vi "main_ctrl.vi"(8 "error in":errorcluster) -> (0 "error out":errorcluster caption="Error")   [LabVIEW 2013]
uses:
  <vilib>/Rock Robotics/WPI/DriverStation/WPI_DriverStationRobotMode2.ctl
  typedefs/Test/test data.ctl
  typedefs/Test/test controls.ctl
  typedefs/fg_typedef.ctl
  typedefs/Vision/vision enable.ctl
  typedefs/Vision/vision data.ctl
  typedefs/State Machine/subStates.ctl
  typedefs/State Machine/singleUseSubstate.ctl
  <vilib>/Rock Robotics/WPI/Solenoid/WPI_SolenoidValue.ctl
  <vilib>/Rock Robotics/WPI/Compressor/WPI_CompressorGetSetRefNum.vi
  <vilib>/Rock Robotics/WPI/RobotDrive/WPI_RobotDriveGetSetRefNum.vi
  <vilib>/Rock Robotics/WPI/RobotDrive/WPI_RobotDriveArcadeDrive_Standard(NoSaturation).vi
  <vilib>/Rock Robotics/WPI/Solenoid/WPI_SolenoidSetEnum.vi
  state machine master/Cancel State Machine - Pickup.vi
  state machine master/Cancel State Machine - Load.vi
panel:
  out "vision errors":errorcluster
  in  "Test\nControls":T1={"Drive Train"=0.0, "Arm"=0.0, "Belts"=0.0, "Drive Train"=FALSE, "Arm"=FALSE, "Belts"=FALSE, "Home Arm Encoder"=FALSE, "Home Right Drive Encoder"=FALSE, "Home Left Drive Encoder"=FALSE, "Extend Shooter"=FALSE, "Retract Shooter"=FALSE, "Latch"=FALSE, "Unlatch"=FALSE, "Shift High"=FALSE, "Shift Low"=FALSE, "Compressor"=TRUE} {"Belts" scale=-1.0..1.0; "Arm" scale=-1.0..1.0; "Drive Train" scale=-1.0..1.0}
  out "Test Data":T2={"Light Sensor"=FALSE, "Shooter Up"=TRUE, "Shooter Down"=FALSE, "Left Rate"=0.0, "Left Distance"=0.0, "Right Rate"=0.0, "Right Distance"=0.0, "Rate"=0.0, "Distance"=0.0, "At Distance Limit"=FALSE, "Encoder Failure"=FALSE, "No Rate Read"=FALSE, "Directional Issue"=FALSE, "Latched"=FALSE, "Unlatched"=TRUE, "Shifted High"=FALSE, "Shifted Low"=TRUE, "Extended"=FALSE, "Retracted"=TRUE, "Left - Encoder Failure"=FALSE, "Left - No Rate Read"=FALSE, "Right - Encoder Failure"=FALSE, "Right - No Rate Read"=FALSE, "Charging"=FALSE, "Full"=FALSE, "On/Off"=FALSE, "DisVision"=FALSE, "2 Ball"=FALSE, "HotGoal"=FALSE, "Shoot"=FALSE}
  out "Robot Mode":T3
  out "Vision mSPI":u32
  out "Vision IPS":dbl
  out "Main IPS":dbl
  out "Main mSPI":u32
  # "Test Input/Output"
  # "MAIN CONTROL"
  # "holds robot control code - dual parallel state machine"
  # "SPI: milliseconds per iteration\nIPS: iterations per second"
  # "Pneumatics"
  # "Home Encoders"
  # "Manual Override"
  # "Joystick Control"
  # "Arm Safeties"
  # "Drive Safeties"
  # "Sensors"
  # "Drive Encoders"
  # "Pneumatics Commands"
  # "Compressor"
  # "Auto Config"
  # "Arm Encoder"
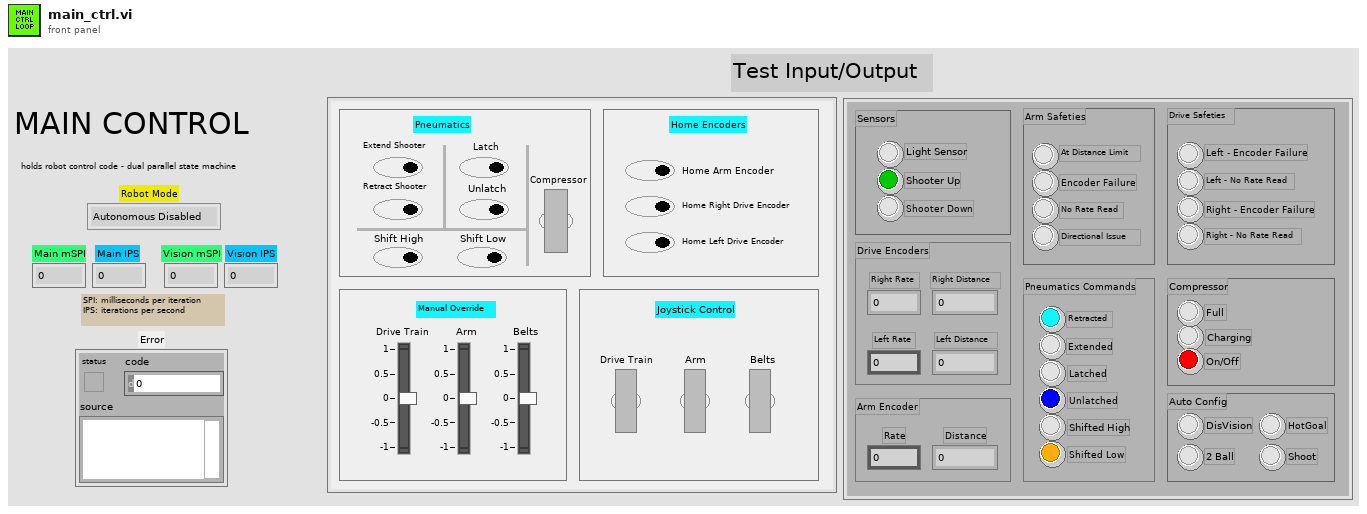
[diagram p1: front panel]
types:
  T1 = typedef "test controls.ctl" = cluster{"Drive Train":dbl, "Arm":dbl, "Belts":dbl, "Drive Train":bool, "Arm":bool, "Belts":bool, "Home Arm Encoder":bool, "Home Right Drive Encoder":bool, "Home Left Drive Encoder":bool, "Extend Shooter":bool, "Retract Shooter":bool, "Latch":bool, "Unlatch":bool, "Shift High":bool, "Shift Low":bool, "Compressor":bool}
  T2 = typedef "test data.ctl" = cluster{"Light Sensor":bool, "Shooter Up":bool, "Shooter Down":bool, "Left Rate":dbl, "Left Distance":dbl, "Right Rate":dbl, "Right Distance":dbl, "Rate":dbl, "Distance":dbl, "At Distance Limit":bool, "Encoder Failure":bool, "No Rate Read":bool, "Directional Issue":bool, "Latched":bool, "Unlatched":bool, "Shifted High":bool, "Shifted Low":bool, "Extended":bool, "Retracted":bool, "Left - Encoder Failure":bool, "Left - No Rate Read":bool, "Right - Encoder Failure":bool, "Right - No Rate Read":bool, "Charging":bool, "Full":bool, "On/Off":bool, "DisVision":bool, "2 Ball":bool, "HotGoal":bool, "Shoot":bool}
  T3 = typedef "WPI_DriverStationRobotMode2.ctl" = enum16{"Autonomous Disabled", "Autonomous Enabled", "Teleop Disabled", "Teleop Enabled", "Timeout", "Finish", "Test Disabled", "Test Enabled"}
  T4 = typedef "fg_typedef.ctl" = enum16{"Get", "Set"}
  T5 = typedef "vision data.ctl" = cluster{"x":dbl, "y":dbl, "area":dbl, "width":dbl, "height":dbl, "Hot Goal Present?":bool, "distance":dbl}
  T6 = typedef "vision enable.ctl" = enum16{"Enable", "Disable", "Stop"}
  T7 = typedef "WPI_CameraDevRef.ctl" = cluster{"Camera Address":string, "CameraStatus":errorcluster, "Acquire Image Notifier":refnum<notifier>}
  T8 = typedef "IMAQ Image.ctl" = refnum<image>
  T9 = cluster{"Vision mSPI":u32, "Main mSPI":u32, "Dash mSPI":u32}
  T10 = typedef "WPI_RobotDriveDevRef.ctl" = cluster{"DevStatus":errorcluster, "Motors[]":T11[], "Square Inputs":bool, "Max Output":dbl, "Isochronous":bool}
  T11 = typedef "WPI_MotorControlDeviceRef.ctl" = cluster{"DeviceStatus":errorcluster, "Type":enum16{"PWM", "CAN"}, "PWM":cluster{"Digital Module":T12, "PWM Channel":T13, "DeadBand":T14}, "CAN":cluster{"Device Number":u8, "Control Mode":T15, "Semaphore":T16, "Max Vout":dbl}, "Invert":bool, "TransformRef":T17, "InvTransformRef":T17}
  T12 = typedef "FPGA_TypedefDigitalModule.ctl" = enum16{"Digital Module 1", "Digital Module 2"}
  T13 = typedef "FPGA_DIOPWMChannel.ctl" = enum8{"PWM 1", "PWM 2", "PWM 3", "PWM 4", "PWM 5", "PWM 6", "PWM 7", "PWM 8", "PWM 9", "PWM 10", "Invalid"}
  T14 = typedef "WPI_PWMDeadband.ctl" = cluster{"Name":string, "maxPositivePwm":i32, "minPositivePwm":i32, "centerPwm":i32, "maxNegativePwm":i32, "minNegativePwm":i32, "angularRange":u16}
  T15 = typedef "WPI_CANJaguar_ControlMode.ctl" = enum8{"Percent VBus", "Current", "Speed", "Position", "Voltage"}
  T16 = typedef "Semaphore RefNum" = refnum<k1>
  T17 = typedef "WPI_PWMTransform_ConPane.ctl" = refnum<vi>
  T18 = typedef "WPI_SolenoidDevRef.ctl" = cluster{"DevStatus":errorcluster, "Solenoid Module":T19, "Forward Solenoid Channel":T20, "Reverse Solenoid Channel":T20}
  T19 = typedef "FPGA_TypedefSolenoidModule.ctl" = enum16{"Solenoid Module 1", "Solenoid Module 2"}
  T20 = typedef "WPI_SolenoidChannel.ctl" = enum8{"Solenoid 1", "Solenoid 2", "Solenoid 3", "Solenoid 4", "Solenoid 5", "Solenoid 6", "Solenoid 7", "Solenoid 8", "Invalid"}
  T21 = typedef "WPI_CompressorDevRef.ctl" = cluster{"DevStatus":errorcluster, "DigitalInputDevRef":T22, "RelayDevRef":T24}
  T22 = typedef "WPI_DigitalInputDevRef.ctl" = cluster{"DevStatus":errorcluster, "DIO Channel":T23, "Digital Module":T12}
  T23 = typedef "FPGA_DIOChannel.ctl" = enum8{"DIO 1", "DIO 2", "DIO 3", "DIO 4", "DIO 5", "DIO 6", "DIO 7", "DIO 8", "DIO 9", "DIO 10", "DIO 11", "DIO 12", "DIO 13", "DIO 14", "Invalid"}
  T24 = typedef "WPI_RelayDevRef.ctl" = cluster{"DevStatus":errorcluster, "Relay Channel":T25, "Digital Module":T12, "Relay Direction":T26}
  T25 = typedef "FPGA_DIORelayChannel.ctl" = enum8{"Relay 1", "Relay 2", "Relay 3", "Relay 4", "Relay 5", "Relay 6", "Relay 7", "Relay 8", "Invalid"}
  T26 = typedef "WPI_RelayDirection.ctl" = enum16{"Both directions", "Forward only", "Reverse only"}
  T27 = typedef "WPI_SolenoidValue.ctl" = enum16{"Off", "On", "Forward", "Reverse"}
  T28 = typedef "subStates.ctl" = enum16{"null", "wait", "driver control", "auto", "manual override", "hold position", "rotate", "pickup", "pass", "recover pass", "load", "goto shoot", "shoot high goal", "shoot low goal", "cancel arm", "cancel shooter", "end", "test"}
  T29 = typedef "singleUseSubstate.ctl" = enum16{"null", "wait", "shift high", "shift low", "extend shooter", "retract shooter", "latch", "unlatch", "end"}
  T30 = typedef "WPI_DriverStationMatch Info.ctl" = cluster{"Autonomous Elapsed Seconds":dbl, "TeleOp Elapsed Seconds":dbl, "Disabled Elapsed Seconds":dbl, "Visited Autonomous":bool, "Visited TeleOp":bool, "Visited Disabled":bool, "Autonomous Settings":cluster{"Autonomous Style":enum16{"Iterative", "Independent"}, "VI Refnum":refnum<vi>}}
  T31 = typedef "WPI_DriverStationDerivedRobotMode.ctl" = enum16{"Init", "Execute", "Stop"}
  T32 = typedef "Loop 2 Datatype.ctl" = cluster{"State":T28, "Waiting Loop":i32, "State to Wait For":i32, "Loop ID":i32, "Exit Value":i32, "Joystick Y":dbl, "Joystick Z":dbl}
  T33 = typedef "Loop 1 Datatype.ctl" = cluster{"State":T28, "Waiting Loop":i32, "State to Wait For":i32, "Loop ID":i32, "Exit Value":i32}
  T34 = typedef "Loop 3 Datatype.ctl" = cluster{"State":T28, "Waiting Loop":i32, "State to Wait For":i32, "Loop ID":i32, "Exit Value":i32, "Joystick Y":dbl, "Tune Setpoint":cluster{"Increment":bool, "Decrement":bool}}
  T35 = typedef "Loop 0 Datatype.ctl" = cluster{"State":T28, "Waiting Loop":i32, "State to Wait For":i32, "Loop ID":i32, "Exit Value":i32, "X Axis":dbl, "Y Axis":dbl, "Z Axis":dbl}
  T36 = typedef "dashboard safety status data.ctl" = cluster{"At Distance Limit":bool, "No Rate Read":bool, "Encoder Failure":bool, "Encoder Directional Issue":bool}
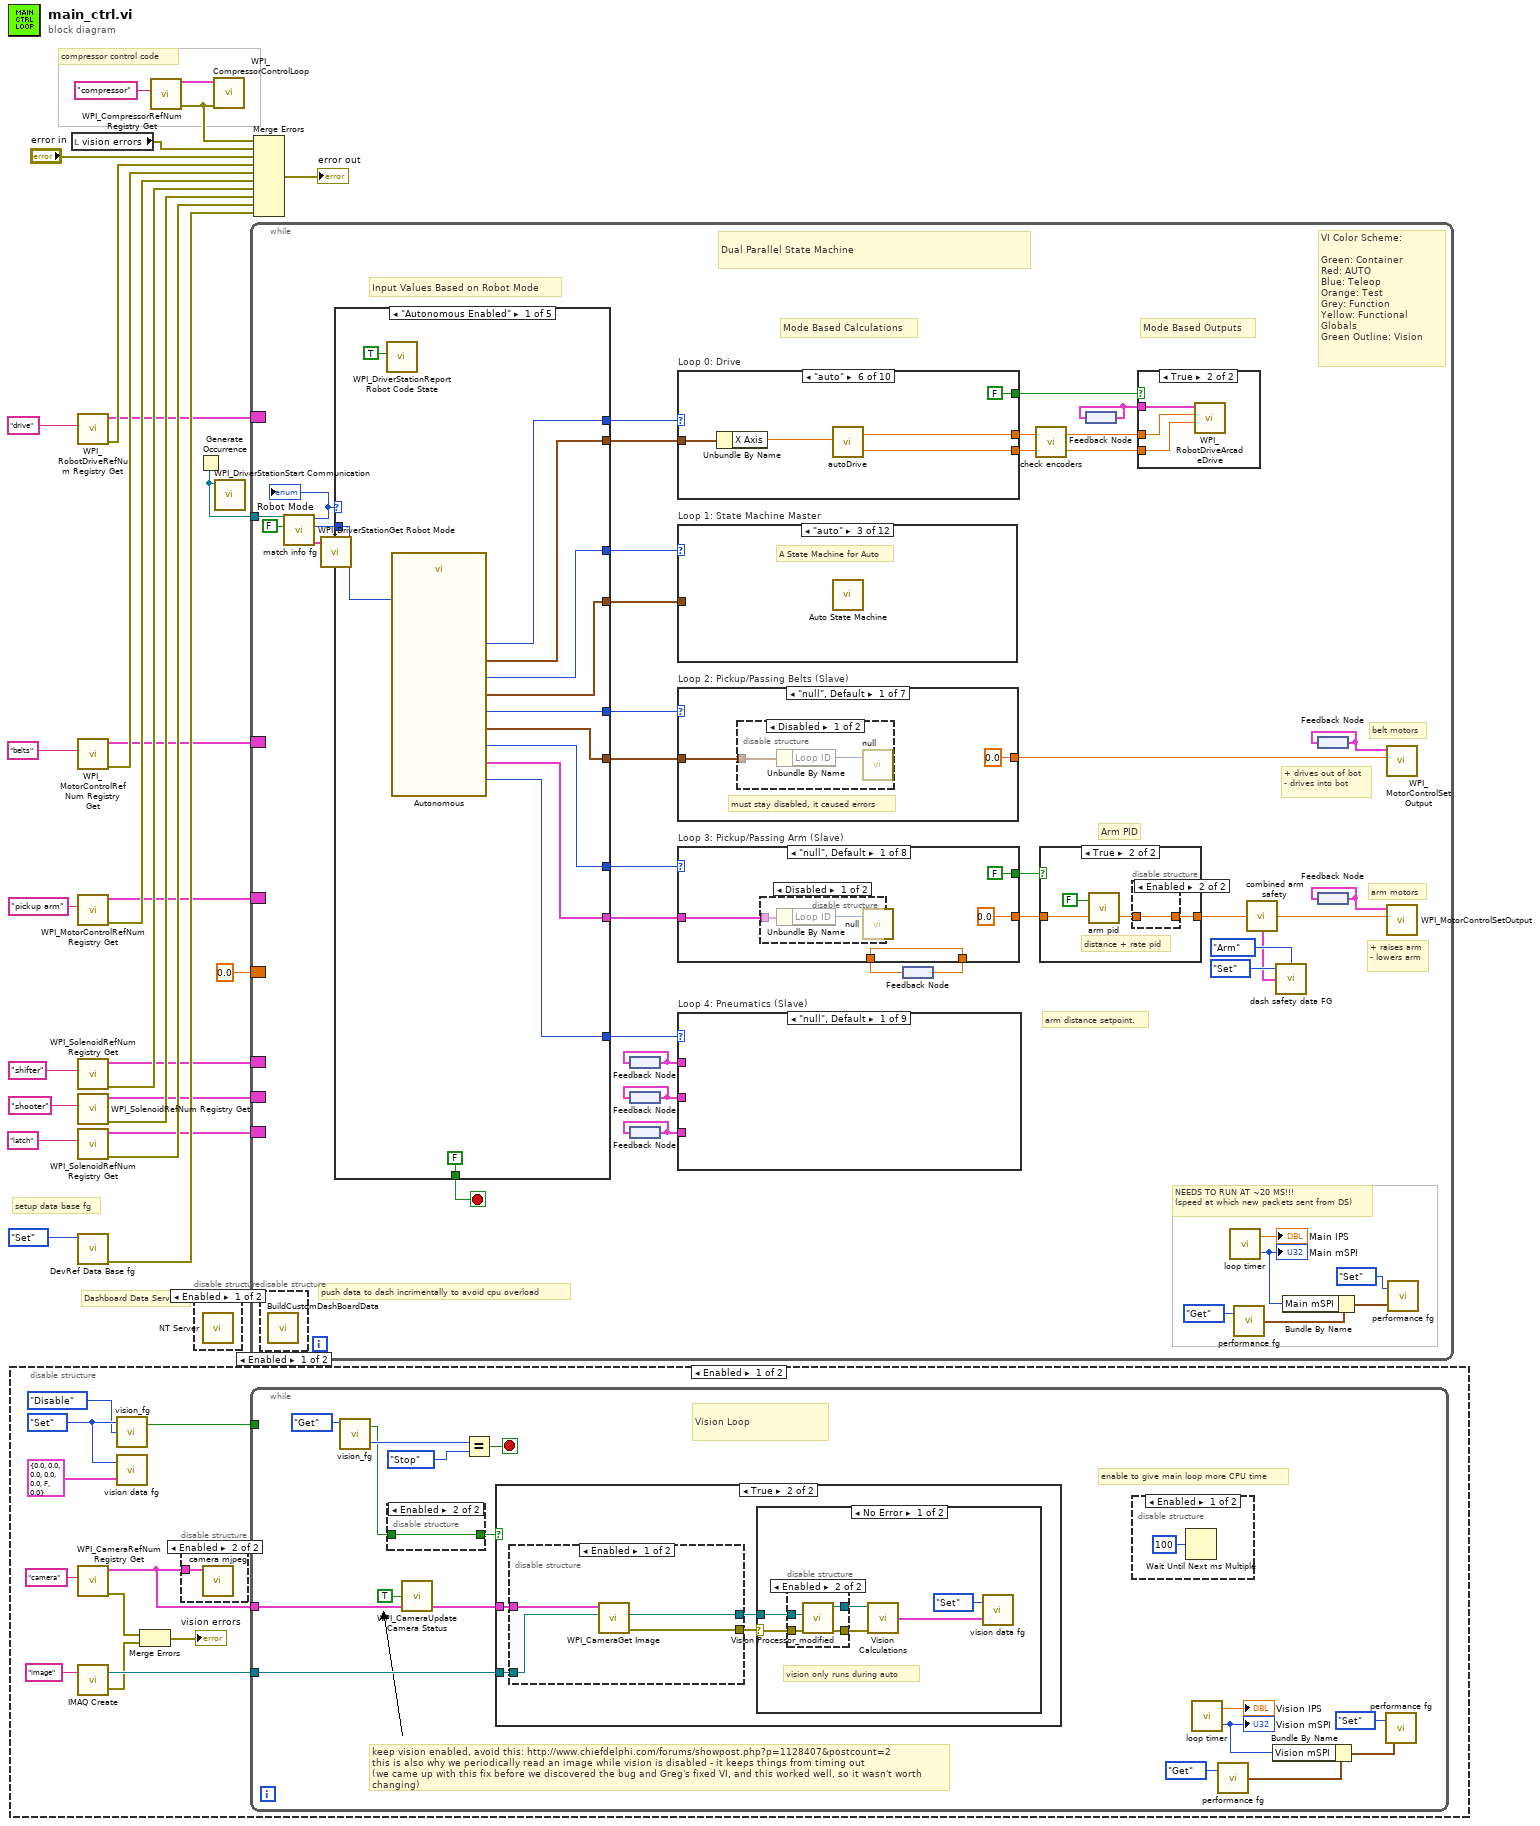
[diagram p0: block diagram]
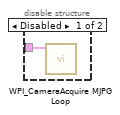
[diagram p3: hidden frame]
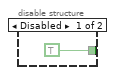
[diagram p4: hidden frame]
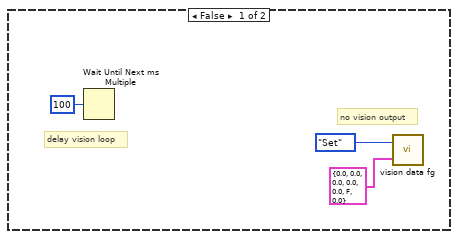
[diagram p6: hidden frame]
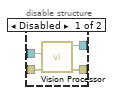
[diagram p7: hidden frame]
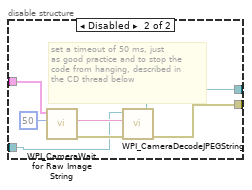
[diagram p9: hidden frame]
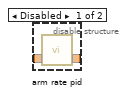
[diagram p12: hidden frame]
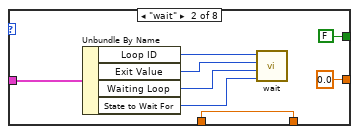
[diagram p14: hidden frame]
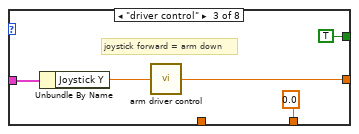
[diagram p15: hidden frame]
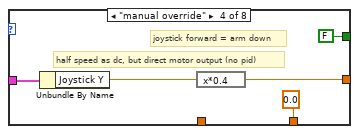
[diagram p16: hidden frame]
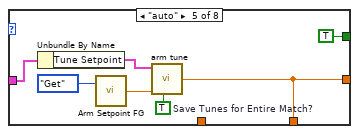
[diagram p17: hidden frame]
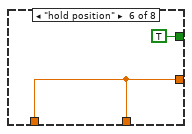
[diagram p18: hidden frame]
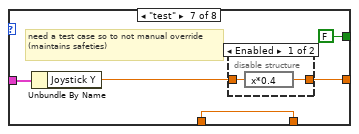
[diagram p19: hidden frame]
diagram:
  # "compressor control code"
  # "Dashboard Data Server"
  # "setup data base fg"
  n1 = disable-structure shown="Enabled" {
    frame Enabled {
      w37 = fg_typedef."Set" ("Enum")
      n2 = call <vilib>:"WPI_CameraRefNum Registry Get.vi"("refnum name"="camera") -> ("error out"=w30:errorcluster, "CameraDevRef"=w34:T7)  [unwired: 9 in]
      n3 = call "IMAQ Create"("Image Name"="image") -> ("New Image"=w39:T8, "error out"=w31:errorcluster)  [unwired: 4 in]
      n4 = call "vision_fg.vi"("Action"=vision_enable."Disable", "Menu"=w37) -> ("Enabled?"=w38:bool)  [unwired: 1 in, 1 out]
      n5 = call "vision data fg.vi"("Input"=T5 {"x"=0.0, "y"=0.0, "area"=0.0, "width"=0.0, "height"=0.0, "Hot Goal Present?"=FALSE, "distance"=0.0} ("Cluster"), "Menu"=w37) -> ()  [unwired: 1 out]
      n6 = Merge Errors(w30, w31) -> (→"vision errors":errorcluster)
      n7 = disable-structure shown="Enabled" {
        disable-tunnel: w34 -> [w40 w41]
        frame Disabled {
          n8 = call <vilib>:"WPI_CameraAcquire MJPG Loop.vi"("CameraDevRef"=w40) -> ()  [unwired: 11 in]
        }
        frame Enabled {
          n9 = call "camera mjpeg.vi"("CameraDevRef"=w41) -> ()  [unwired: 11 in]
        }
      }
      n10 = while {
        tunnel: w39 -> [w56]
        tunnel: w34 -> [w55]
        tunnel: w38 -> [_]
        stop <- w57 stop-if-true
        # "keep vision enabled, avoid this: http://www.chiefdelphi.com/forums/showpost.php?p=1128407&postcount=2\nthis is also why we periodically read an image while vision is disabled - it keeps things from timing out\n(we came up with this fix before we discovered the bug and Greg's fixed VI, and this worked well, so it wasn't worth changing)"
        # "enable to give main loop more CPU time"
        # "Vision Loop"
        n11 = call "vision_fg.vi"("Menu"=fg_typedef."Get" ("Enum")) -> ("State Out"=w51:T6, "Enabled?"=w42:bool)  [unwired: 2 in]
        n12 = disable-structure shown="Enabled" {
          disable-tunnel: [TRUE w59] -> w43
          disable-tunnel: w42 -> [_ w59]
          frame Disabled {
          }
          frame Enabled {
          }
        }
        n13 = call <vilib>:"WPI_CameraUpdate Camera Status.vi"("CameraDevRef In"=w55, "Enable Vision"=TRUE) -> ("CameraDevRef Out"=w54:T7)  [unwired: 3 in]
        n14 = Equal?(x=w51, y=vision_enable."Stop") -> (x = y?=w57:bool)
        n15 = case shown="True" w43 {
          tunnel: w56 -> [_ w67]
          tunnel: w54 -> [_ w66]
          frame False {
            # "no vision output"
            # "delay vision loop"
            n16 = Wait Until Next ms Multiple(millisecond multiple=u32 100) -> ()  [unwired: 1 out]
            n17 = call "vision data fg.vi"("Input"=T5 {"x"=0.0, "y"=0.0, "area"=0.0, "width"=0.0, "height"=0.0, "Hot Goal Present?"=FALSE, "distance"=0.0} ("Cluster"), "Menu"=fg_typedef."Set" ("Enum")) -> ()  [unwired: 1 out]
          }
          frame True {
            n18 = disable-structure shown="Enabled" {
              disable-tunnel: w67 -> [w84 w88]
              disable-tunnel: w66 -> [w85 w90]
              disable-tunnel: [w83 w87] -> w65
              disable-tunnel: [w82 w86] -> w64
              frame Enabled {
                n19 = call <vilib>:"WPI_CameraGet Image.vi"("Image"=w84, "CameraDevRef"=w85) -> ("error out"=w82:errorcluster, "Image Out"=w83:T8)  [unwired: 7 in, 1 out]
              }
              frame Disabled {
                # "set a timeout of 50 ms, just\nas good practice and to stop the \ncode from hanging, described in \nthe CD thread below"
                n20 = call <vilib>:"WPI_CameraWait for Raw Image String.vi"("Timeout in ms (-1)"=50, "CameraDevRef"=w90) -> ("error out"=w92:errorcluster, "String"=w91:string)  [unwired: 3 in, 5 out]
                n21 = call <vilib>:"WPI_CameraDecodeJPEGString.vi"("error in"=w92, "Compressed Image"=w91, "Image In"=w88) -> ("error out"=w86:errorcluster, "Image Out"=w87:T8)  [unwired: 3 out]
              }
            }
            n22 = case shown="No Error" w64 {
              selector: w64 -> [w72 _]
              tunnel: w65 -> [w71 _]
              frame No Error {
                # "vision only runs during auto"
                n23 = disable-structure shown="Enabled" {
                  disable-tunnel: w72 -> [w77 w80]
                  disable-tunnel: w71 -> [w76 w81]
                  disable-tunnel: [w75 w78] -> w70
                  disable-tunnel: [w74 w79] -> w69
                  frame Disabled {
                    n24 = call "Vision Processor.vi"("error in"=w77, "Image In"=w76) -> ("error out"=w74:errorcluster, "Image Out"=w75:T8)  [unwired: 5 in]
                  }
                  frame Enabled {
                    n25 = call "Vision Processor_modified.vi"("error in"=w80, "Image In"=w81) -> ("error out"=w79:errorcluster, "Image Out"=w78:T8)  [unwired: 5 in]
                  }
                }
                n26 = call "Vision Calculations.vi"("Image In"=w70, "error in"=w69) -> ("Vision Data"=w68:T5)  [unwired: 3 in]
                n27 = call "vision data fg.vi"("Input"=w68, "Menu"=fg_typedef."Set" ("Enum")) -> ()  [unwired: 1 out]
              }
              frame Error {
              }
            }
          }
        }
        n28 = disable-structure shown="Enabled" {
          frame Enabled {
            n29 = Wait Until Next ms Multiple(millisecond multiple=u32 100) -> ()  [unwired: 1 out]
          }
          frame Disabled {
          }
        }
        n30 = call "loop timer.vi"() -> ("IPS"=→"Vision IPS":dbl, "SPI"=w49:u32)  [unwired: 1 in]
        "Vision mSPI" <- w49
        n31 = call "performance fg.vi"("Menu"=fg_typedef."Get") -> ("Output"=w47:T9)  [unwired: 1 in]
        n32 = Bundle By Name(cluster=w47, "Vision mSPI"=w49) -> (w46:T9)
        n33 = call "performance fg.vi"("Input"=w46, "Menu"=fg_typedef."Set") -> ()  [unwired: 1 out]
      }
    }
    frame Disabled {
      # "vision disabled"
    }
  }
  n34 = local read "vision errors"() -> (w1:errorcluster)
  n35 = call <vilib>:"WPI_RobotDriveRefNum Registry Get.vi"("refnum name"="drive") -> ("error out"=w27:errorcluster, "RobotDriveDevRef"=w3:T10)  [unwired: 9 in]
  n36 = call <vilib>:"WPI_MotorControlRefNum Registry Get.vi"("refnum name"="belts") -> ("error out"=w26:errorcluster, "MotorControlDevRef"=w7:T11)  [unwired: 9 in]
  n37 = call <vilib>:"WPI_MotorControlRefNum Registry Get.vi"("refnum name"="pickup arm") -> ("error out"=w25:errorcluster, "MotorControlDevRef"=w10:T11)  [unwired: 9 in]
  n38 = call <vilib>:"WPI_SolenoidRefNum Registry Get.vi"("refnum name"="shifter") -> ("error out"=w24:errorcluster, "SolenoidDevRef"=w17:T18)  [unwired: 9 in]
  n39 = call <vilib>:"WPI_SolenoidRefNum Registry Get.vi"("refnum name"="shooter") -> ("error out"=w23:errorcluster, "SolenoidDevRef"=w5:T18)  [unwired: 9 in]
  n40 = call <vilib>:"WPI_SolenoidRefNum Registry Get.vi"("refnum name"="latch") -> ("error out"=w22:errorcluster, "SolenoidDevRef"=w6:T18)  [unwired: 9 in]
  n41 = call "DevRef Data Base fg.vi"("Menu"=fg_typedef."Set") -> ("error out"=w28:errorcluster)  [unwired: 2 in, 8 out]
  n42 = call <vilib>:"WPI_CompressorRefNum Registry Get.vi"("refnum name"="compressor") -> ("error out"=w2:errorcluster, "CompressorDevRef"=w18:T21)  [unwired: 9 in]
  n43 = disable-structure shown="Enabled" {
    frame Enabled {
      n44 = call <vilib>:"NT Server.vi"() -> ()  [unwired: 12 in]
    }
    frame Disabled {
    }
  }
  n45 = Generate Occurrence() -> (w15:refnum<k4>)
  n46 = call <vilib>:"WPI_CompressorControlLoop.vi"("error in (no error)"=w2, "CompressorDevRef"=w18) -> ()  [unwired: 10 in]
  n47 = call <vilib>:"WPI_DriverStationStart Communication.vi"("occurrence"=w15) -> ()  [unwired: 11 in]
  n48 = while {
    tunnel: w15 -> [w116]
    border: w3 -> [_]
    border: w17 -> [_]
    border: w6 -> [_]
    border: w5 -> [_]
    border: w7 -> [_]
    border: w10 -> [_]
    border: 0.0 ("setpoint") -> [_]
    stop <- w131 stop-if-true
    # "Arm PID"
    # "Mode Based Outputs"
    # "arm motors"
    # "arm distance setpoint."
    # "push data to dash incrimentally to avoid cpu overload"
    # "+ raises arm\n- lowers arm"
    # "+ drives out of bot\n- drives into bot"
    # "belt motors"
    # "VI Color Scheme:\n\nGreen: Container\nRed: AUTO\nBlue: Teleop\nOrange: Test \nGrey: Function\nYellow: Functional Globals\nGreen Outline: Vision"
    # "Input Values Based on Robot Mode"
    # "Mode Based Calculations"
    # "NEEDS TO RUN AT ~20 MS!!!\n(speed at which new packets sent from DS)"
    # "Dual Parallel State Machine"
    n49 = disable-structure shown="Enabled" {
      frame Enabled {
        n50 = call "BuildCustomDashBoardData.vi"() -> ()  [unwired: 12 in]
      }
      frame Disabled {
      }
    }
    n51 = call <vilib>:"WPI_DriverStationGet Robot Mode.vi"("Finish"=FALSE, "DS Occurrence"=w116) -> ("Match Info out"=w99:T30, "Call Context"=w115:T31, "Robot Mode"=w114:T3)  [unwired: 7 out]
    "Robot Mode" <- w114
    n52 = call "match info fg.vi"("Match Info"=w99) -> ()  [unwired: 26 in, 1 out]
    n53 = case shown="\"Autonomous Enabled\"" w114 {
      tunnel: [w321 w336 w345 w353 w359] -> w118
      tunnel: w115 -> [w314 w332 w348 _ _]
      tunnel: [w319 w335 w347 w353 w359] -> w133
      tunnel: [w315 w333 w339 singleUseSubstate."null" ("SubState 5") singleUseSubstate."end" ("SubState 5")] -> w132
      tunnel: [FALSE FALSE FALSE FALSE TRUE] -> w131
      tunnel: [w323 w331 w343 w353 w359] -> w108
      tunnel: [w322 w330 w344 _ _] -> w125
      tunnel: [w320 w329 w346 _ _] -> w124
      tunnel: [w318 w328 w342 _ _] -> w123
      tunnel: [w316 w327 w340 _ _] -> w121
      tunnel: [w317 w326 w341 w353 w359] -> w107
      frame "Autonomous Enabled" {
        n54 = call <vilib>:"WPI_DriverStationReport Robot Code State.vi"("Autonomous"=TRUE) -> ()  [unwired: 10 in, 1 out]
        n55 = call "Autonomous.vi"("Call Context"=w314) -> ("SubState 2"=w319:T28, "Loop 2 Data"=w318:T32, "SubState 1"=w321:T28, "Loop 1 Data"=w320:T33, "Loop 3 Data"=w316:T34, "SubState 0"=w323:T28, "SubState 3"=w317:T28, "Loop 0 Data"=w322:T35, "SubState 4"=w315:T29)  [unwired: 2 in]
      }
      frame "Teleop Enabled" {
        n56 = call <vilib>:"WPI_DriverStationReport Robot Code State.vi"("TeleOp"=TRUE) -> ()  [unwired: 10 in, 1 out]
        n57 = call "Teleop.vi"("Call Context"=w332) -> ("SubState 3"=w326:T28, "SubState 4"=w333:T29, "Loop 3 Data"=w327:T34, "SubState 0"=w331:T28, "Loop 1 Data"=w329:T33, "Loop 0 Data"=w330:T35, "SubState 1"=w336:T28, "Loop 2 Data"=w328:T32, "SubState 2"=w335:T28)  [unwired: 10 in]
      }
      frame "Test Enabled" {
        n58 = call <vilib>:"WPI_DriverStationReport Robot Code State.vi"("Test"=TRUE) -> ()  [unwired: 10 in, 1 out]
        n59 = call "Test.vi"("Test Controls"="Test\nControls", "Call Context"=w348) -> ("Loop 2 Data"=w342:T32, "SubState 2"=w347:T28, "Loop 1 Data"=w346:T33, "SubState 1"=w345:T28, "SubState 3"=w341:T28, "Loop 0 Data"=w344:T35, "Loop 3 Data"=w340:T34, "SubState 0"=w343:T28, "SubState 4"=w339:T29, "Test Data"=→"Test Data":T2)
      }
      frame "Autonomous Disabled", "Teleop Disabled", "Timeout", "Test Disabled" {
        w353 = subStates."null" ("SubState 0")
        # "set all loops to null"
        # "make sure to disable vision\nwe don't need it here"
        # "robot disabled, timeout"
        n60 = call <vilib>:"WPI_DriverStationReport Robot Code State.vi"("Disabled"=TRUE) -> ()  [unwired: 10 in, 1 out]
        n61 = call "vision_fg.vi"("Action"=vision_enable."Disable", "Menu"=fg_typedef."Set") -> ()  [unwired: 1 in, 2 out]
      }
      frame "Finish" {
        w359 = subStates."end" ("Loop State")
        # "Stop All Loops"
        # "stop the while loop"
        # "stop DS comms"
        # "stop vision loop"
        n62 = call <vilib>:"WPI_DriverStationStop Communication.vi"("StopCommunication"=TRUE) -> ()  [unwired: 10 in, 1 out]
        n63 = call "vision_fg.vi"("Action"=vision_enable."Stop", "Menu"=fg_typedef."Set") -> ()  [unwired: 1 in, 2 out]
      }
    }
    n64 = feedback #1() -> (w122:T18)
    n65 = feedback-in #1(w122) -> ()
    n66 = feedback #2() -> (w110:T18)
    n67 = feedback-in #2(w110) -> ()
    n68 = feedback #3() -> (w109:T18)
    n69 = feedback-in #3(w109) -> ()
    n70 = case "Loop 0: Drive" shown="\"auto\"" w108 {
      tunnel: w125 -> [w221 w226 w236 w248 w256 w259 w265 _ w278 _]
      tunnel: [w220 w225 w235 w245 w253 w261 w267 w269 0.0 ("X Axis") w280] -> w96
      tunnel: [w220 w225 w234 w244 w252 w260 w266 w268 w277 w280] -> w95
      tunnel: [FALSE FALSE TRUE FALSE FALSE FALSE FALSE FALSE TRUE FALSE] -> w120
      frame "null", Default {
        w220 = 0.0 ("X Axis")
        n71 = disable-structure shown="Disabled" {
          disable-tunnel: w221 -> [w223 _]
          frame Disabled {
            n72 = Unbundle By Name(w223) -> ("Loop ID"=w222:i32)
            n73 = call "null.vi"("This Loop ID"=w222) -> ()  [unwired: 2 in]
          }
          frame Enabled {
          }
        }
      }
      frame "wait" {
        w225 = 0.0 ("X Axis")
        n74 = Unbundle By Name(w226) -> ("Loop ID"=w230:i32, "Exit Value"=w229:i32, "Waiting Loop"=w228:i32, "State to Wait For"=w227:i32)
        n75 = call "wait.vi"("State to wait for"=w227, "Waiting Loop ID"=w228, "time (ms)"=w229, "Current Loop ID"=w230) -> ()  [unwired: 1 out]
      }
      frame "driver control" {
        n76 = Unbundle By Name(w236) -> ("X Axis"=w232:dbl, "Y Axis"=w233:dbl)
        n77 = disable-structure shown="Enabled" {
          disable-tunnel: w232 -> [w240 w242]
          disable-tunnel: w233 -> [w239 w241]
          disable-tunnel: [w238 w242] -> w235
          disable-tunnel: [w237 w241] -> w234
          frame Disabled {
            n78 = call "calc arcade drive pwm.vi"("Y axis value"=w239, "X axis value"=w240) -> ("Right Speed"=w237:dbl, "Left Speed"=w238:dbl)  [unwired: 1 in, 1 out]
          }
          frame Enabled {
          }
        }
      }
      frame "manual override" {
        n79 = Unbundle By Name(w248) -> ("X Axis"=w247:dbl, "Y Axis"=w246:dbl)
        n80 = expression code="x/2"(w247) -> (w245:dbl)
        n81 = expression code="x/2"(w246) -> (w244:dbl)
      }
      frame "hold position" {
        n82 = Unbundle By Name(w256) -> ("X Axis"=w255:dbl, "Y Axis"=w254:dbl)
        n83 = call "closed drive.vi"("Acrade Drive?"=TRUE, "Y axis value (Left)"=w254, "X axis value (Right)"=w255, "Threshold (.4)"=0.4) -> ("right"=w252:dbl, "left"=w253:dbl)
      }
      frame "auto" {
        n84 = Unbundle By Name(w259) -> ("X Axis"=w257:dbl)
        n85 = call "autoDrive.vi"("Distance"=w257) -> ("right speed"=w260:dbl, "left speed"=w261:dbl)  [unwired: 2 in, 1 out]
      }
      frame "rotate" {
        n86 = Unbundle By Name(w265) -> ("X Axis"=w264:dbl, "Y Axis"=w263:dbl)
        n87 = call "rotate.vi"("Rate"=w263, "Angle"=w264) -> ("right speed"=w266:dbl, "left speed"=w267:dbl)  [unwired: 1 in, 1 out]
      }
      frame "goto shoot" {
        n88 = disable-structure shown="Enabled" {
          disable-tunnel: [w272 _] -> w269
          disable-tunnel: [w271 _] -> w268
          frame Disabled {
            # "consider implimenting closed hold with drive"
            n89 = call "vision data fg.vi"("Menu"=fg_typedef."Get") -> ("Output"=w273:T5)  [unwired: 1 in]
            n90 = call "goto location.vi"("Image Data"=w273) -> ("left speed"=w272:dbl, "right speed"=w271:dbl)
          }
          frame Enabled {
            # "not going to do this"
          }
        }
      }
      frame "test" {
        n91 = Unbundle By Name(w278) -> ("Y Axis"=w277:dbl)
      }
      frame "end" {
        w280 = 0.0 ("X Axis")
      }
    }
    n92 = case "Loop 1: State Machine Master" shown="\"auto\"" w118 {
      tunnel: w124 -> [w298 w299 _ _ _ _ _ _ _ _ _ _]
      frame "null", Default {
        n93 = Unbundle By Name(w298) -> ("Loop ID"=w297:i32)
        n94 = call "null.vi"("This Loop ID"=w297) -> ()  [unwired: 2 in]
      }
      frame "wait" {
        n95 = Unbundle By Name(w299) -> ("Loop ID"=w303:i32, "Exit Value"=w302:i32, "Waiting Loop"=w301:i32, "State to Wait For"=w300:i32)
        n96 = call "wait.vi"("State to wait for"=w300, "Waiting Loop ID"=w301, "time (ms)"=w302, "Current Loop ID"=w303) -> ()  [unwired: 1 out]
      }
      frame "auto" {
        # "A State Machine for Auto"
        n97 = call "Auto State Machine.vi"() -> ()  [unwired: 12 in]
      }
      frame "manual override" {
        w309 = FALSE ("Can Shoot Safely?")
        w304 = TRUE ("exit in")
        # "Manual Shoot"
        n98 = call "single use states FG.vi"("exit in"=w304, "substate"=singleUseSubstate."unlatch", "menu (get)"=enum16{"set", "get"}."set") -> ()  [unwired: 5 in, 4 out]
        n99 = call "states FG.vi"("exit in"=w304, "subState in"=subStates."null", "menu (get)"=enum16{"set", "get"}."set", "Loop ID"=1) -> ()  [unwired: 4 in, 4 out]
        n100 = call "safe shoot error.vi"("Can Shoot Safely?"=w309, "Menu"=fg_typedef."Set") -> ()  [unwired: 1 out]
        n101 = call "arm during load cancel.vi"("Arm Canceled During Load?"=w309, "Mode"=enum16{"Get", "Set", "Teleop Set"}."Set") -> ()  [unwired: 1 out]
      }
      frame "pickup" {
        # "A State Machine for Pickup"
        n102 = call "Pickup State Machine.vi"() -> ()  [unwired: 12 in]
      }
      frame "pass" {
        # "A State Machine for Passing"
        n103 = call "Pass State Machine.vi"() -> ()  [unwired: 12 in]
      }
      frame "recover pass" {
        # "If a pass fails i.e. ball gets stuck, let the drivers fix it"
        # "A State Machine for Recovering a Pass"
        n104 = call "Pass Recovery State Machine.vi"() -> ()  [unwired: 12 in]
      }
      frame "load" {
        # "ball can now (after this) be high or low goal shot"
        # "A State Machine for Loading"
        n105 = call "Load State Machine.vi"() -> ()  [unwired: 12 in]
      }
      frame "shoot high goal" {
        # "A State Machine for High Goal Shooting"
        n106 = call "Shoot High Goal State Machine.vi"() -> ()  [unwired: 12 in]
      }
      frame "shoot low goal" {
        # "A State Machine for Low Goal Shooting"
        n107 = call "Shoot Low Goal State Machine.vi"() -> ()  [unwired: 12 in]
      }
      frame "cancel arm" {
        # "A State Machine for Canceling Pickup"
        n108 = call-poly "Cancel State Machine - Polymorphic.vi"() -> ()  [unwired: 1 in]
      }
      frame "cancel shooter" {
        # "A State Machine for Canceling Load"
        n109 = call-poly "Cancel State Machine - Polymorphic.vi"() -> ()  [unwired: 1 in]
      }
    }
    n110 = case "Loop 2: Pickup/Passing Belts (Slave)" shown="\"null\", Default" w133 {
      tunnel: w123 -> [w188 w192 w199 w202 w209 w211 _]
      tunnel: [0.0 ("output") 0.0 ("output") w197 w200 w206 w210 0.0 ("Joystick Y")] -> w111
      frame "null", Default {
        # "must stay disabled, it caused errors"
        n111 = disable-structure shown="Disabled" {
          disable-tunnel: w188 -> [w190 _]
          frame Disabled {
            n112 = Unbundle By Name(w190) -> ("Loop ID"=w189:i32)
            n113 = call "null.vi"("This Loop ID"=w189) -> ()  [unwired: 2 in]
          }
          frame Enabled {
          }
        }
      }
      frame "wait" {
        n114 = Unbundle By Name(w192) -> ("Loop ID"=w196:i32, "Exit Value"=w195:i32, "Waiting Loop"=w194:i32, "State to Wait For"=w193:i32)
        n115 = call "wait.vi"("State to wait for"=w193, "Waiting Loop ID"=w194, "time (ms)"=w195, "Current Loop ID"=w196) -> ()  [unwired: 1 out]
      }
      frame "driver control" {
        # "which joystick? should be specified in name."
        # "joystick forward = out of bot"
        n116 = Unbundle By Name(w199) -> ("Joystick Y"=w198:dbl)
        n117 = Negate(x=w198) -> (-x=w197:dbl)
      }
      frame "manual override" {
        # "essentially driver control, but 1/2 speed?"
        # "joystick forward = out of bot"
        n118 = Unbundle By Name(w202) -> ("Joystick Y"=w201:dbl)
        n119 = expression code="-x/2"(w201) -> (w200:dbl)
      }
      frame "auto" {
        # "get speed to go as set by master and tune"
        n120 = Unbundle By Name(w209) -> ("Joystick Z"=w207:dbl)
        n121 = call "Joystick tuner.vi"("Joystick Z"=w207, "Loop ID"=2) -> ("Output"=w205:dbl)  [unwired: 7 in]
        n122 = call "Belt Speed FG.vi"("Menu"=fg_typedef."Get") -> ("Speed Out"=w204:dbl)  [unwired: 1 in]
        n123 = Multiply(x=w205, y=w204) -> (x*y=w206:dbl)
      }
      frame "test" {
        n124 = Unbundle By Name(w211) -> ("Joystick Y"=w210:dbl)
      }
      frame "end" {
      }
    }
    n125 = case "Loop 4: Pneumatics (Slave)" shown="\"null\", Default" w132 {
      tunnel: w122 -> [_ _ w282 w283 _ _ _ _ _]
      tunnel: w110 -> [_ _ _ _ w285 w287 _ _ w295]
      tunnel: w109 -> [_ _ _ _ _ _ w289 w291 w293]
      frame "null", Default {
      }
      frame "wait" {
      }
      frame "shift high" {
        n126 = call-poly <vilib>:"WPI_SolenoidSet.vi"("Value"=WPI_SolenoidValue."Forward", "SolenoidDevRef"=w282) -> ()  [unwired: 8 in, 2 out]
      }
      frame "shift low" {
        n127 = call-poly <vilib>:"WPI_SolenoidSet.vi"("Value"=WPI_SolenoidValue."Reverse", "SolenoidDevRef"=w283) -> ()  [unwired: 8 in, 2 out]
      }
      frame "extend shooter" {
        n128 = call-poly <vilib>:"WPI_SolenoidSet.vi"("Value"=WPI_SolenoidValue."Forward", "SolenoidDevRef"=w285) -> ()  [unwired: 8 in, 2 out]
      }
      frame "retract shooter" {
        n129 = call-poly <vilib>:"WPI_SolenoidSet.vi"("Value"=WPI_SolenoidValue."Reverse", "SolenoidDevRef"=w287) -> ()  [unwired: 8 in, 2 out]
      }
      frame "latch" {
        # "When the latch piston\nis reversed, the latch\nis closed. When the\nlatch piston is\nextended, the latch is\nopen."
        n130 = call-poly <vilib>:"WPI_SolenoidSet.vi"("Value"=WPI_SolenoidValue."Reverse", "SolenoidDevRef"=w289) -> ()  [unwired: 8 in, 2 out]
      }
      frame "unlatch" {
        # "When the latch piston\nis reversed, the latch\nis closed. When the\nlatch piston is\nextended, the latch is\nopen."
        n131 = call-poly <vilib>:"WPI_SolenoidSet.vi"("Value"=WPI_SolenoidValue."Forward", "SolenoidDevRef"=w291) -> ()  [unwired: 8 in, 2 out]
      }
      frame "end" {
        # "retract shooter and unlatch"
        n132 = call-poly <vilib>:"WPI_SolenoidSet.vi"("Value"=WPI_SolenoidValue."Reverse", "SolenoidDevRef"=w295) -> ()  [unwired: 8 in, 2 out]
        n133 = call-poly <vilib>:"WPI_SolenoidSet.vi"("Value"=WPI_SolenoidValue."Forward", "SolenoidDevRef"=w293) -> ()  [unwired: 8 in, 2 out]
      }
    }
    n134 = feedback #4() -> (w102:dbl)
    n135 = case "Loop 3: Pickup/Passing Arm (Slave)" shown="\"null\", Default" w107 {
      tunnel: w121 -> [w146 w152 w160 w166 w173 _ w180 _]
      tunnel: [FALSE FALSE TRUE FALSE TRUE TRUE FALSE FALSE] -> w105
      tunnel: [0.0 ("output") 0.0 ("output") w159 w164 w167 w174 w176 0.0 ("Joystick Y")] -> w104
      tunnel: [w143 w149 0.0 ("setpoint") 0.0 ("setpoint") w167 w174 w177 w184] -> w103
      tunnel: w102 -> [w143 w149 _ _ _ w174 w177 w184]
      frame "null", Default {
        n136 = disable-structure shown="Disabled" {
          disable-tunnel: w146 -> [w148 _]
          frame Disabled {
            n137 = Unbundle By Name(w148) -> ("Loop ID"=w147:i32)
            n138 = call "null.vi"("This Loop ID"=w147) -> ()  [unwired: 2 in]
          }
          frame Enabled {
          }
        }
      }
      frame "wait" {
        n139 = Unbundle By Name(w152) -> ("Loop ID"=w156:i32, "Exit Value"=w155:i32, "Waiting Loop"=w154:i32, "State to Wait For"=w153:i32)
        n140 = call "wait.vi"("State to wait for"=w153, "Waiting Loop ID"=w154, "time (ms)"=w155, "Current Loop ID"=w156) -> ()  [unwired: 1 out]
      }
      frame "driver control" {
        # "joystick forward = arm down"
        n141 = Unbundle By Name(w160) -> ("Joystick Y"=w158:dbl)
        n142 = call "arm driver control.vi"("Joystick Y"=w158) -> ("Setpoint"=w159:dbl)
      }
      frame "manual override" {
        # "half speed as dc, but direct motor output (no pid)"
        # "joystick forward = arm down"
        n143 = Unbundle By Name(w166) -> ("Joystick Y"=w165:dbl)
        n144 = expression code="x*0.4"(w165) -> (w164:dbl)
      }
      frame "auto" {
        w168 = TRUE  # Save Tunes for Entire Match?
        n145 = Unbundle By Name(w173) -> ("Tune Setpoint"=w170:cluster{"Increment":bool, "Decrement":bool})
        n146 = call "Arm Setpoint FG.vi"("Menu"=fg_typedef."Get") -> ("Setpoint Out"=w169:dbl)  [unwired: 1 in]
        n147 = call "arm tune.vi"("Tune Data"=w170, "Setpoint"=w169, "Save Tunes for Entire Match?"=w168) -> ("Tuned Setpoint"=w167:dbl)  [unwired: 4 in]
      }
      frame "hold position" {
      }
      frame "test" {
        # "need a test case so to not manual override\n(maintains safeties)"
        n148 = Unbundle By Name(w180) -> ("Joystick Y"=w179:dbl)
        n149 = disable-structure shown="Enabled" {
          disable-tunnel: w179 -> [w182 w183]
          disable-tunnel: [w181 w183] -> w176
          frame Enabled {
            n150 = expression code="x*0.4"(w182) -> (w181:dbl)
          }
          frame Disabled {
          }
        }
      }
      frame "end" {
      }
    }
    n151 = feedback-in #4(w103) -> ()
    n152 = call "check encoders.vi"("Right (Y)"=w95, "Left (X)"=w96) -> ("Right (Y) Out"=w93:dbl, "Left (X) Out"=w94:dbl)
    n153 = case shown="True" w105 {
      tunnel: w104 -> [w135 w138]
      tunnel: [w135 w136] -> w100
      frame False {
        # "open loop"
      }
      frame True {
        # "distance + rate pid"
        n154 = call "arm pid.vi"("Setpoint"=w138, "Autotune?"=FALSE) -> ("Output"=w137:dbl)  [unwired: 1 in]
        n155 = disable-structure shown="Enabled" {
          disable-tunnel: w137 -> [w141 w142]
          disable-tunnel: [w140 w142] -> w136
          frame Disabled {
            n156 = call "arm rate pid.vi"("Rate In"=w141) -> ("Rate Out"=w140:dbl)  [unwired: 2 in]
          }
          frame Enabled {
          }
        }
      }
    }
    n157 = feedback #5() -> (w119:T10)
    n158 = feedback-in #5(w119) -> ()
    n159 = case shown="True" w120 {
      tunnel: w94 -> [w214 w218]
      tunnel: w93 -> [w213 w217]
      tunnel: w119 -> [w215 w216]
      frame False {
        n160 = call <vilib>:"WPI_RobotDriveMotors.vi"("RightSpeed"=w213, "LeftSpeed"=w214, "RobotDriveDevRef"=w215) -> ()  [unwired: 6 in, 3 out]
      }
      frame True {
        n161 = call-poly <vilib>:"WPI_RobotDriveArcadeDrive.vi"("Y axis value"=w217, "X axis value"=w218, "RobotDriveDevRef"=w216) -> ()  [unwired: 6 in, 3 out]
      }
    }
    n162 = call "loop timer.vi"() -> ("IPS"=→"Main IPS":dbl, "SPI"=w130:u32)  [unwired: 1 in]
    "Main mSPI" <- w130
    n163 = call "performance fg.vi"("Menu"=fg_typedef."Get") -> ("Output"=w127:T9)  [unwired: 1 in]
    n164 = call "combined arm safety.vi"("Input"=w100) -> ("Safe Output"=w106:dbl, "Safety Data"=w97:T36)  [unwired: 13 in]
    n165 = call "dash safety data FG.vi"("Mechanism"=enum16{"Arm", "Drive Train"}."Arm", "Arm Safety Data"=w97, "Menu"=fg_typedef."Set") -> ()  [unwired: 1 in, 2 out]
    n166 = Bundle By Name(cluster=w127, "Main mSPI"=w130) -> (w126:T9)
    n167 = feedback #6() -> (w113:T11)
    n168 = feedback-in #6(w113) -> ()
    n169 = feedback #7() -> (w112:T11)
    n170 = feedback-in #7(w112) -> ()
    n171 = call <vilib>:"WPI_MotorControlSetOutput.vi"("Output"=w111, "MotorControlDevRef"=w113) -> ()  [unwired: 7 in, 3 out]
    n172 = call <vilib>:"WPI_MotorControlSetOutput.vi"("Output"=w106, "MotorControlDevRef"=w112) -> ()  [unwired: 7 in, 3 out]
    n173 = call "performance fg.vi"("Input"=w126, "Menu"=fg_typedef."Set") -> ()  [unwired: 1 out]
  }
  n174 = Merge Errors(w2, w1, "error in", w27, w26, w25, w24, w23, w22, w28) -> (→"error out":errorcluster)
